vi "disable module.vi"(8 "error in":errorcluster, 9 "timeout (-1)":i32=-1, 10 "Module ID":string, 11 "Standard Engine Runtime in":refnum<class "Standard Engine Runtime.lvclass">) -> (0 "error out":errorcluster, 3 "Standard Engine Runtime out":refnum<class "Standard Engine Runtime.lvclass">)   [LabVIEW 2013, in "Standard Engine Runtime.lvclass"]
uses:
  Standard Engine Runtime.lvclass
  main engine/message request type.ctl
  main engine/main engine.lvlib
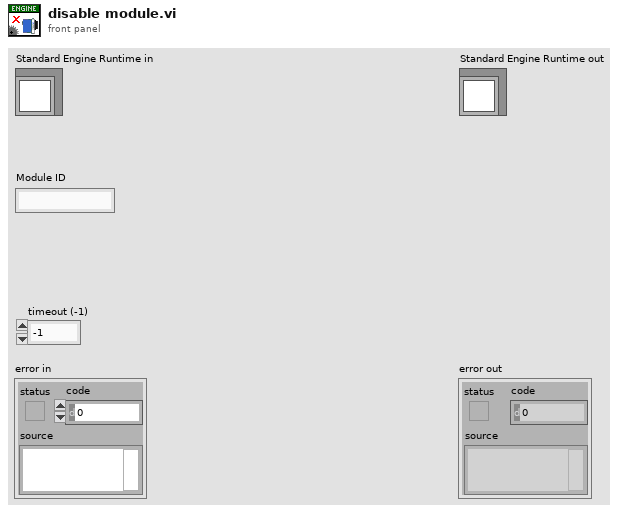
[diagram p1: front panel]
types:
  T1 = typedef "main engine.lvlib/message request type.ctl" = enum8{"set value", "disable module", "enable module"}
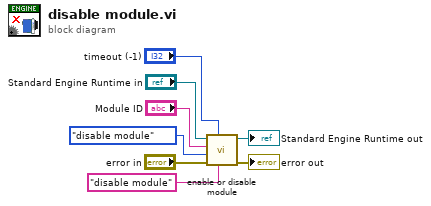
[diagram p0: block diagram]
diagram:
  n1 = call "enable or disable module.vi"("source"="disable module", "timeout"="timeout (-1)", "error in (no error)"="error in", "request type"=message_request_type."disable module", "Module ID"="Module ID", "Standard Engine Runtime in"="Standard Engine Runtime in") -> ("error out"=→"error out":errorcluster, "Standard Engine Runtime out"=→"Standard Engine Runtime out":refnum<class "Standard Engine Runtime.lvclass">)  [unwired: 4 in]
